vi "Fix Angles.vi"(1 "Input Angles":T1) -> (0 "Output Angles":T1)   [LabVIEW 2018]
uses:
  Encoder Data.ctl
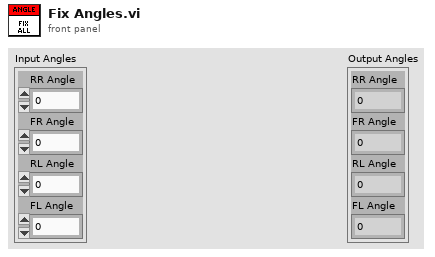
[diagram p1: front panel]
types:
  T1 = typedef "Encoder Data.ctl" = cluster{"RR Angle":dbl, "FR Angle":dbl, "RL Angle":dbl, "FL Angle":dbl}
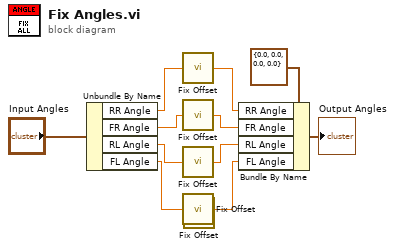
[diagram p0: block diagram]
diagram:
  n1 = Unbundle By Name("Input Angles") -> ("RR Angle"=w2:dbl, "FR Angle"=w5:dbl, "RL Angle"=w9:dbl, "FL Angle"=w6:dbl)
  n2 = call "Fix Offset.vi"("Input Angle"=w2) -> ("Output Angle"=w3:dbl)
  n3 = call "Fix Offset.vi"("Input Angle"=w5) -> ("Output Angle"=w4:dbl)
  n4 = call "Fix Offset.vi"("Input Angle"=w9) -> ("Output Angle"=w8:dbl)
  n5 = call "Fix Offset.vi"("Input Angle"=w6) -> ("Output Angle"=w7:dbl)
  n6 = call "Fix Offset.vi"() -> ()  [unwired: 1 in, 1 out]
  n7 = Bundle By Name(cluster=T1 {"RR Angle"=0.0, "FR Angle"=0.0, "RL Angle"=0.0, "FL Angle"=0.0} ("Input Angles 2"), "RR Angle"=w3, "FR Angle"=w4, "RL Angle"=w8, "FL Angle"=w7) -> (→"Output Angles":T1)
